vi "Actor Core.vi"(8 "error in":errorcluster, 11 "Lock-in in":refnum<class "Lock-in.lvclass">) -> (0 "error out":errorcluster, 3 "Actor out":refnum<class "Actor.lvclass">)   [LabVIEW 2015, in "Lock-in.lvclass"]
doc: "(<B>Filename</B>: Actor Framework.lvlib:Actor.lvclass:Actor Core.vi)\n\nReceives messages to the actor, reacts to them, and initiates any error handling that may shut the actor down.\n\nDescendant classes may override this VI to append parallel tasks for the actor to complete while it handles messages. Overrides use the Call Parent Method node."
uses:
  Lock-in.lvclass
  <vilib>/ActorFramework/Actor/Actor.lvclass
  NHMFL_Core/Libraries/Instruments/Instrument Driver/Lock-in Driver/Lock-in Configuration.ctl
  Measure_core/Measure Object/Measure Object.lvclass/Measure Object.ctl
  <vilib>/ActorFramework/Actor/Actor.lvclass/Actor.ctl
  <vilib>/ActorFramework/Message Enqueuer/Message Enqueuer.lvclass/Message Enqueuer.ctl
  Lock-in Messages/Set Frequency Msg/Set Frequency Msg.lvclass/Set Frequency Msg.ctl
  Measure_core/Measure Object/Read stop event.vi
  <vilib>/ActorFramework/Message Enqueuer/Init from Existing Queue.vi
  <vilib>/ActorFramework/Message Enqueuer/Enqueue.vi
  <vilib>/ActorFramework/Message Priority Queue/Priority Enqueue.vi
  Measure_core/Instrument Recorders/Instrument Recorder/Instrument Recorder.lvclass
  <vilib>/ActorFramework/Message Enqueuer/Message Enqueuer.lvclass
  Lock-in Messages/Set Frequency Msg/Set Frequency Msg.lvclass
panel:
  in  "Configuration":T1 {"Time constant" format="%#_6ps"; "Frequency" format="%#_6pHz"}
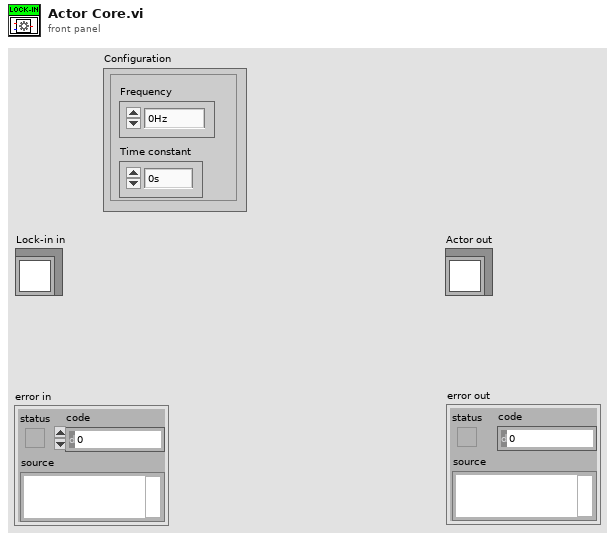
[diagram p1: front panel]
types:
  T1 = typedef "Lock-in Configuration.ctl" = cluster{"Frequency":dbl, "Time constant":dbl}
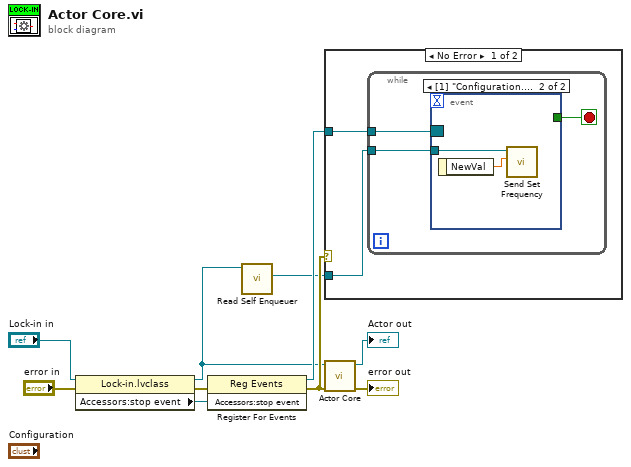
[diagram p0: block diagram]
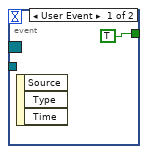
[diagram p2: hidden frame]
diagram:
  n1 = property class="Lock-in.lvclass"(reference="Lock-in in", error in="error in") -> (reference out=w2:refnum<class "Lock-in.lvclass">, error out=w4:errorcluster, "Accessors:stop event"=w7:refnum<user-event>)
  n2 = register-events(error in=w4, w7) -> (reference out=w6:refnum<event-registration>, error out=w3:errorcluster)  [unwired: 1 in]
  n3 = call <vilib>:"Read Self Enqueuer.vi"("Actor"=w2) -> ("Self Enqueuer"=w1:refnum<class "Message Enqueuer.lvclass">)  [unwired: 10 in]
  n4 = case shown="No Error" w3 {
    tunnel: w6 -> [w12 _]
    tunnel: w1 -> [w11 _]
    frame No Error {
      n5 = while {
        tunnel: w12 -> [w15]
        tunnel: w11 -> [w13]
        stop <- w14 stop-if-true
        n6 = event shown="[1] \"Configuration.Frequency\": Value Change" {
          selector: w15 -> [_ _]
          dyn-events: _ -> [_ _]
          timeout: _ -> [_ _]
          tunnel: [TRUE _] -> w14
          tunnel: w13 -> [_ w18]
          event User Event {
            n7 = event-data() -> ()  [unwired: 1 in, 3 out]
          }
          event Value Change {
            n8 = event-data() -> ("NewVal"=w17:dbl)  [unwired: 1 in]
            n9 = call "Send Set Frequency.vi"("Frequency"=w17, "Message Enqueuer"=w18) -> ()  [unwired: 8 in, 2 out]
          }
        }
      }
    }
    frame Error {
    }
  }
  n10 = call-parent "Actor Core.vi"("error in"=w3, "Measure Object in"=w2) -> ("error out"=→"error out":errorcluster, "Actor out"=→"Actor out":refnum<class "Actor.lvclass">)  [unwired: 8 in]
